vi "AutoCorrelation (single).vi"(8 "error in (no error)":errorcluster, 11 "XY-data a":cluster{"X-array":dbl[], "Y-array":dbl[]} {"Y-array" format="%.2p"; "X-array" format="%.2p"}) -> (0 "error out":errorcluster, 3 "XY-data a out":cluster{"X-array":dbl[], "Y-array":dbl[]} {"Y-array" format="%.2p"; "X-array" format="%.2p"})   [LabVIEW 2019, in "xy_utilities.lvlib"]
doc: "Compute the autocorrelation <b>R_aa</b> of <b>XY-data a</b>."
uses:
  xy_utilities.lvlib
  <vilib>/Analysis/2dsp.llb/1D Auto Correlation (DBL).vi
  <vilib>/Analysis/NI_AALPro.lvlib
panel:
  out "R_aa":cluster{"X-array":dbl[], "Y-array":dbl[]} {"Y-array" format="%.2p"; "X-array" format="%.2p"}
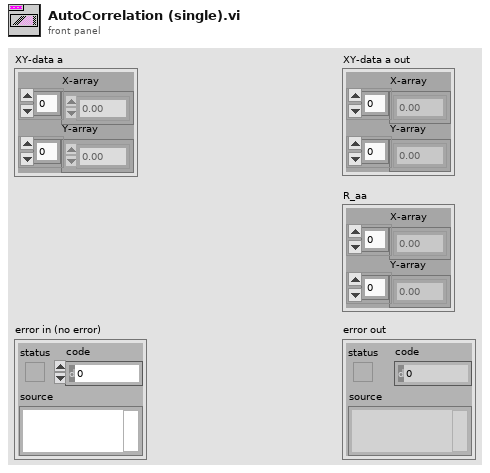
[diagram p1: front panel]
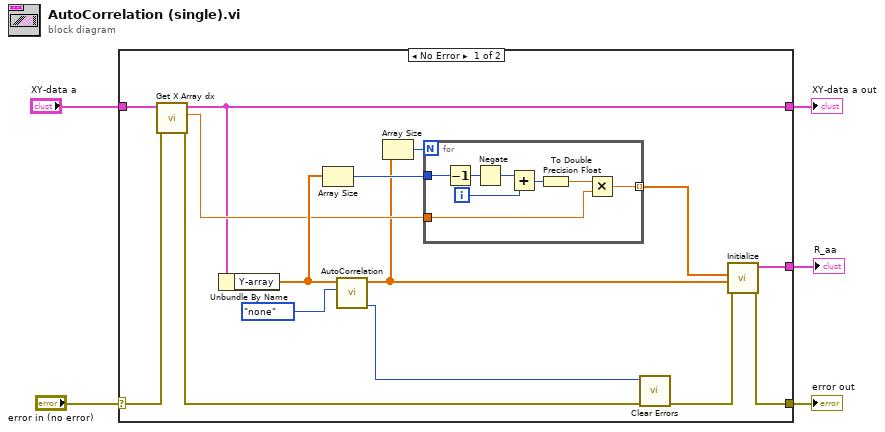
[diagram p0: block diagram]
diagram:
  n1 = case shown="No Error" "error in (no error)" {
    selector: "error in (no error)" -> [w16 w30]
    tunnel: [w7 w30] -> w4
    tunnel: "XY-data a" -> [w17 w29]
    tunnel: [w11 w29] -> w2
    tunnel: [w6 _] -> w1
    frame No Error {
      n2 = call "Get X Array dx.vi"("error in (no error)"=w16, "XY-data"=w17) -> ("error out"=w15:errorcluster, "dX"=w13:dbl, "XY-data out"=w11:cluster{"X-array":dbl[], "Y-array":dbl[]})  [unwired: 6 in, 1 out]
      n3 = Unbundle By Name(w11) -> ("Y-array"=w20:dbl[])
      n4 = Array Size(array=w20) -> (size(s)=w19:i32)
      n5 = call-poly <vilib>:"AutoCorrelation.vi"("normalization"=enum32{"none", "unbiased", "biased"}."none", "X"=w20) -> ("error"=w14:i32, "Rxx"=w9:dbl[])  [unwired: 8 in]
      n6 = Array Size(array=w9) -> (size(s)=w18:i32)
      n7 = for {
        N: w18 -> [_]
        tunnel: w19 -> [w28]
        tunnel: [w24] -> w10 mode=indexing
        tunnel: w13 -> [w22]
        i -> [w26]
        n8 = Decrement(x=w28) -> (x-1=w27:i32)
        n9 = Negate(x=w27) -> (-x=w23:i32)
        n10 = Add(x=w23, y=w26) -> (x+y=w25:i32)
        n11 = To Double Precision Float(number=w25) -> (double precision float=w21:dbl)
        n12 = Multiply(x=w21, y=w22) -> (x*y=w24:dbl)
      }
      n13 = call <vilib>:"Clear Errors.vi"("error in (no error)"=w15, "specific error code to clear (0: all)"=w14) -> ("error out"=w8:errorcluster)  [unwired: 4 in, 1 out]
      n14 = call "Initialize.vi"("error in (no error)"=w8, "Y-array"=w9, "X-array"=w10) -> ("error out"=w7:errorcluster, "XY-data out"=w6:cluster{"X-array":dbl[], "Y-array":dbl[]})  [unwired: 7 in]
    }
    frame Error {
    }
  }
  "error out" <- w4
  "XY-data a out" <- w2
  "R_aa" <- w1
